vi "CSGaussmeterGUI.panel.vi"() -> ()   [LabVIEW 2014, in "CSGaussmeterGUI.lvlib"]
doc: "This is the VI template for the Gaussmeter class."
uses:
  CSGaussmeterGUI.lvlib
  instr.lib/FH_55/TypeDef/Display.ctl
  instr.lib/FH_55/TypeDef/Unit.ctl
  instr.lib/FH_55/TypeDef/Temp_Unit.ctl
  instr.lib/FH_55/TypeDef/Max.ctl
  instr.lib/FH_55/TypeDef/Range.ctl
  instr.lib/FH_55/TypeDef/Unit2.ctl
  CS_Core/CSSystem/CoreDefs/CoreDefs.rawDataType.ctl
  CS_Core/CSSystem/CoreLib/CoreLib.short 2 byte array.vi
  CS_Core/CSSystem/CoreLib/CoreLib.double 2 byte array.vi
  CS_Core/CSSystem/CoreLib/CoreLib.string 2 byte array.vi
  CSGaussmeter/CSGaussmeter.lvlib
  CS_Core/CSSystem/CoreLib/CoreLib.lvlib
  CS_Core/BaseProcess/BaseProcess.lvlib
  CS_Core/CSSystem/CSSystemLib/CSSystemLib.lvlib
  CSlibraries/UtilityLib/UtilityLib.lvlib
  CS_Core/CSObj/CSObj.lvlib
  CS_Core/GUIs/GOGUserGUIs/DeviceBaseGUI/DeviceBaseGUI.lvlib
  instr.lib/FH_55/FH 55.lvlib
panel:
  in  "object ref":refnum<vi>
  out "Messwerte 2":string
  out "status abc":string
  out "status TF":bool
  in  "Stop":bool
  in  "Lesen":bool
  in  "Cluster":cluster{"String":string, "byteArray":T1}
  in  "error out 2":errorcluster
  in  "Control":T7 {"Lower"."Numeric" format="%#_4f"; "Set_Rel"."Numeric" format="%#_4f"; "UPPER"."Numeric" format="%#_4f"}
  in  "Messwerte":cluster{"Numeric":i32, "OK Button":bool}={"Numeric"=1, "OK Button"=FALSE} {"Numeric" min=1}
  out "FH 55 Gauss-/Teslameter":T8
  out "error out":errorcluster
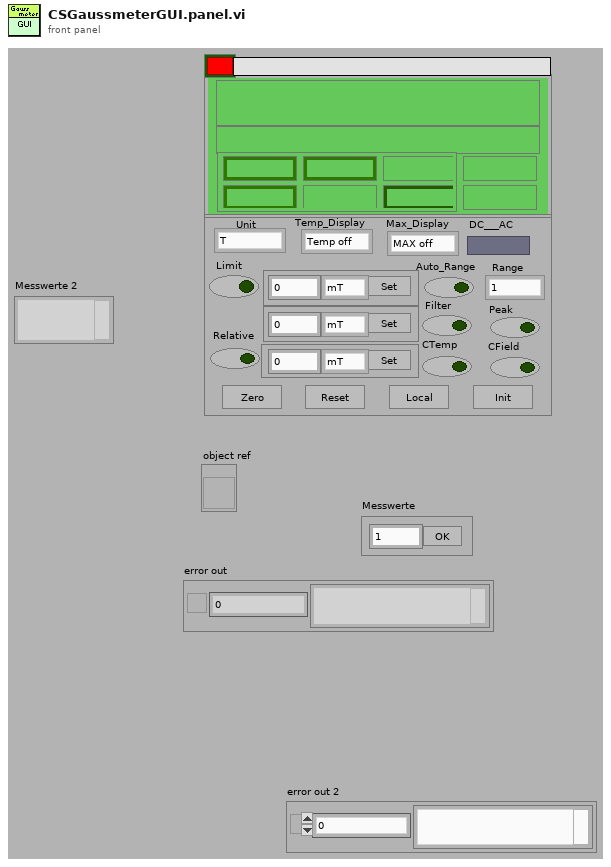
[diagram p1: front panel]
types:
  T1 = typedef "CoreDefs.rawDataType.ctl" = i8[]
  T2 = typedef "FH 55.lvlib/Unit.ctl" = enum16{"T", "G", "A/m"}
  T3 = typedef "FH 55.lvlib/Temp_Unit.ctl" = enum16{"Temp off", "Celsius", "Fahrenheit"}
  T4 = typedef "FH 55.lvlib/Max.ctl" = enum16{"MAX off", "Show MAX", "MAX/MIN"}
  T5 = typedef "FH 55.lvlib/Range.ctl" = enum16{"1", "2", "3", "4", "5", "6", "7"}
  T6 = typedef "FH 55.lvlib/Unit2.ctl" = enum16{"mT", "G", "kA/m"}
  T7 = cluster{" Limit":bool, "Unit":T2, "Temp_Display":T3, "Max_Display":T4, " Filter":bool, " Peak":bool, " Auto_Range":bool, "Range":T5, " Relative":bool, " CTemp":bool, " CField":bool, "DC___AC ":bool, "Lower":cluster{"Numeric":dbl, "Cancel Button":bool, "Unit":T6}, "UPPER":cluster{"Numeric":dbl, "Cancel Button":bool, "Unit":T6}, "Set_Rel":cluster{"Numeric":dbl, "Cancel Button":bool, "Unit":T6}, "Zero":bool, "Reset":bool, " Local":bool, "Init ":bool}
  T8 = typedef "FH 55.lvlib/Display.ctl" = cluster{"current value":string, "Limit":string, "Remote":string, "function ":string, "Cluster":cluster{"AC/DC":string, "Auto":string, "Filter":string, "Range":string, "Rel":string, "Peak":string}}
  T9 = typedef "DeviceBaseGUI.lvlib/DeviceBaseGUI.i attribute.ctl" = cluster{"GOGFrontPanel.i attribute":T10}
  T10 = typedef "GOGFrontPanel.lvlib/GOGFrontPanel.i attribute.ctl" = cluster{"GOGObject":string, "Object":string, "Method":string, "Descriptor":T11, "Input Descriptor":string, "Output Descriptor":string, "inputNames":string[], "outputNames":string[], "Values":cluster{"descriptor":string, "value":string}[]}
  T11 = typedef "BaseProcess.lvlib/BaseProcess.descriptor string definition.ctl" = string
  T12 = typedef "CSGaussmeter.lvlib/CSGaussmeter.i attribute.ctl" = cluster{"Name":string, "VISA Resource Name":refnum<visa-resource-name>, "actValues":cluster{" Limit":bool, "Unit ":T2, "Temp_Unit":T3, "Max":T4, " Filter":bool, " Peak":bool, " Auto_Range":bool, "Range":T5, " Rel":bool, " CTemp":bool, " CField":bool, "AC_DC ":bool, "Set_lower":cluster{"Numeric":dbl, "Cancel Button":bool, "Unit":T6}, "Set_upper":cluster{"Numeric":dbl, "Cancel Button":bool, "Unit":T6}, "Set_Rel":cluster{"Numeric":dbl, "Cancel Button":bool, "Unit":T6}, "Zero":bool, " Local":bool, "Reset":bool, " Init":bool}, "FH 55 Gauss-/Teslameter":T8, "MAX_Value":T13, "MIN_Value":T13, "Rel_Value":T13, "Array ":string[], "LIMU":dbl, " LIML":dbl, "Messwerte 2":string, "Messwerte ":cluster{"Numeric":i32, "OK Button":bool}, "serviceID":cluster{"Current ID":i32, "Unit ID":i32, "Temp ID":i32, "Name ID \n":i32, "Visa ID ":i32}, "setValues ":cluster{" Limit":bool, "Unit ":T2, "Temp_Unit":T3, "Max":T4, " Filter":bool, " Peak":bool, " Auto_Range":bool, "Range":T5, " Rel":bool, " CTemp":bool, " CField":bool, "AC_DC ":bool, "Set_lower":cluster{"Numeric":dbl, "Cancel Button":bool, "Unit":T6}, "Set_upper":cluster{"Numeric":dbl, "Cancel Button":bool, "Unit":T6}, "Set_Rel":cluster{"Numeric":dbl, "Cancel Button":bool, "Unit":T6}, "Zero":bool, " Local":bool, "Reset":bool, " Init":bool}}
  T13 = typedef "FH 55.lvlib/Value_String.ctl" = cluster{"Numeric":dbl, "String":string}
  T14 = cluster{" Limit":bool, "Unit ":T2, "Temp_Unit":T3, "Max":T4, " Filter":bool, " Peak":bool, " Auto_Range":bool, "Range":T5, " Rel":bool, " CTemp":bool, " CField":bool, "AC_DC ":bool, "Set_lower":cluster{"Numeric":dbl, "Cancel Button":bool, "Unit":T6}, "Set_upper":cluster{"Numeric":dbl, "Cancel Button":bool, "Unit":T6}, "Set_Rel":cluster{"Numeric":dbl, "Cancel Button":bool, "Unit":T6}, "Zero":bool, " Local":bool, "Reset":bool, " Init":bool}
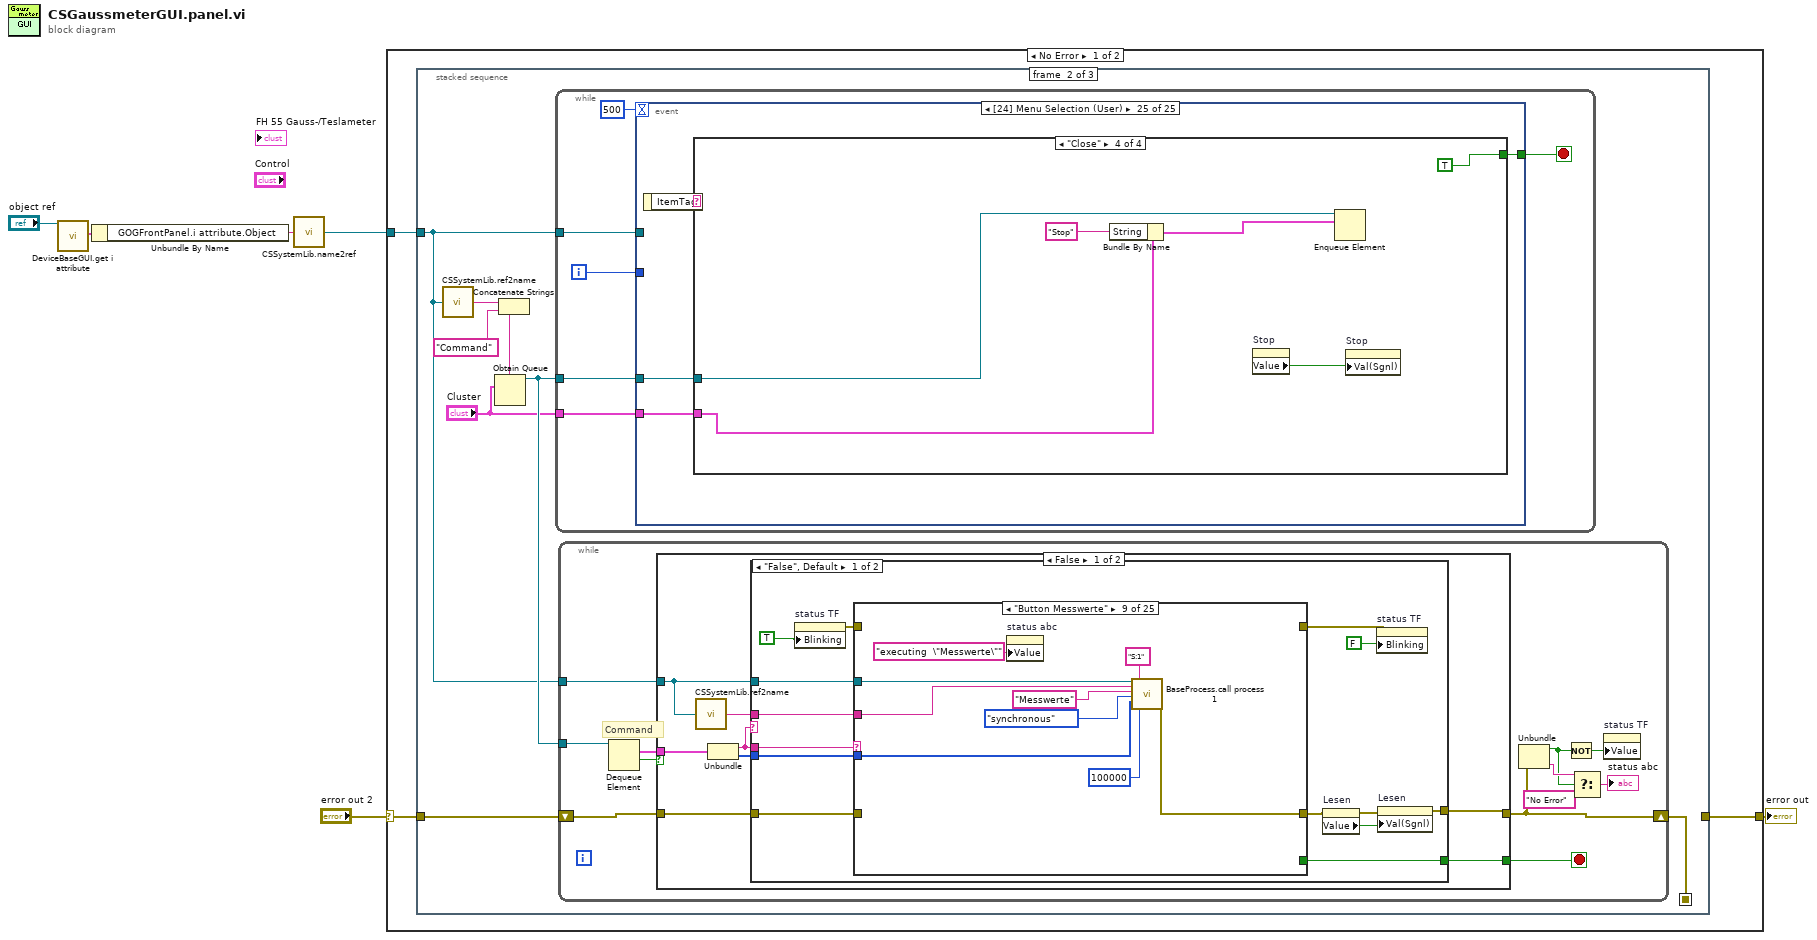
[diagram p0: block diagram]
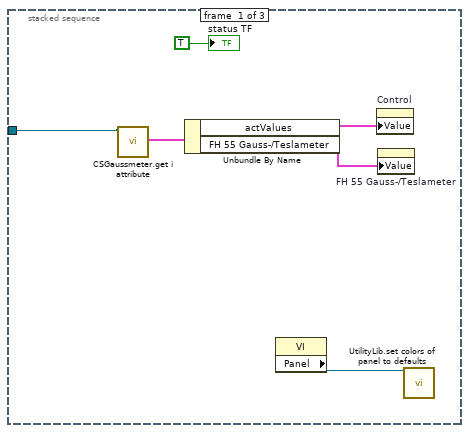
[diagram p2: hidden frame]
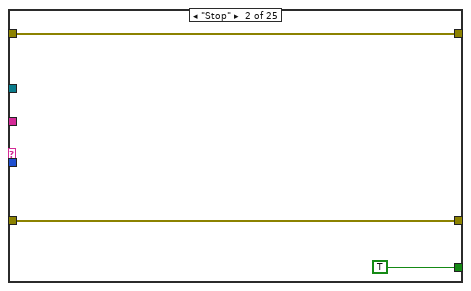
[diagram p4: hidden frame]
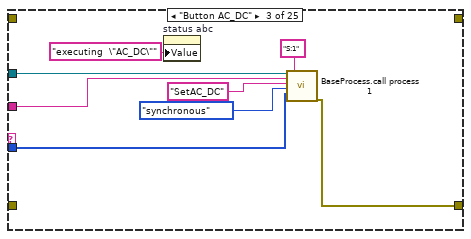
[diagram p5: hidden frame]
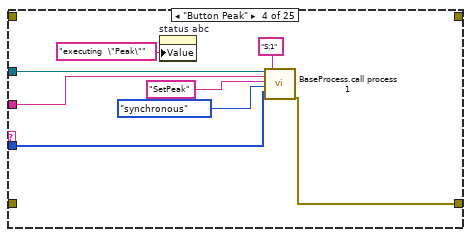
[diagram p6: hidden frame]
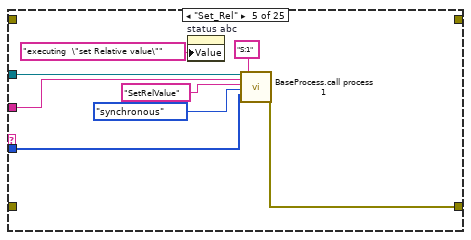
[diagram p7: hidden frame]
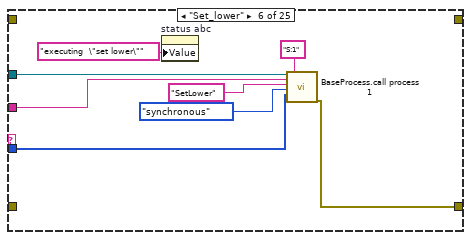
[diagram p8: hidden frame]
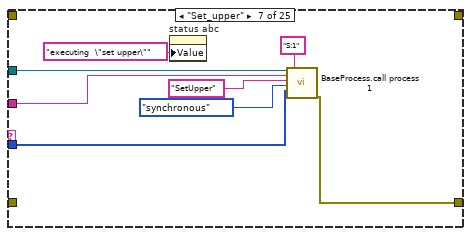
[diagram p9: hidden frame]
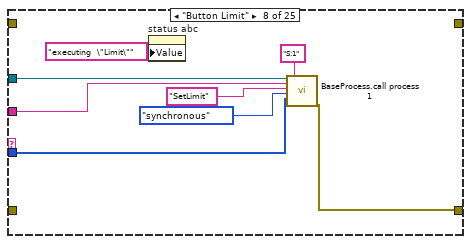
[diagram p10: hidden frame]
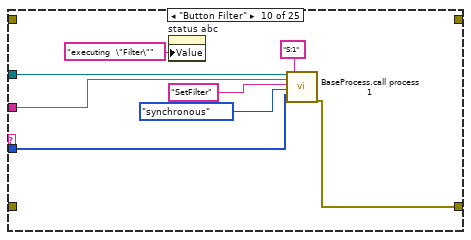
[diagram p11: hidden frame]
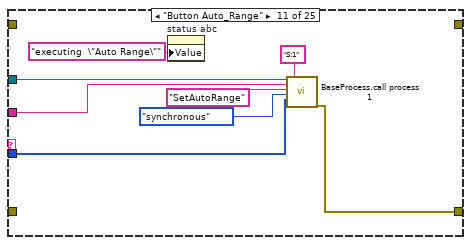
[diagram p12: hidden frame]
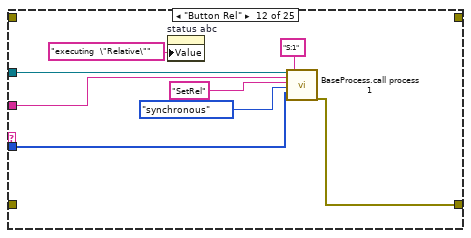
[diagram p13: hidden frame]
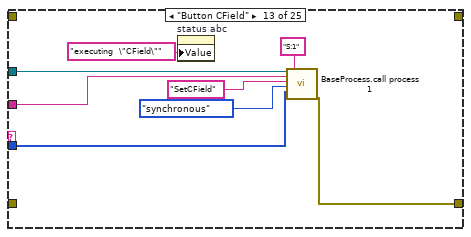
[diagram p14: hidden frame]
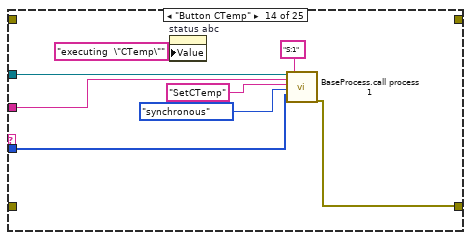
[diagram p15: hidden frame]
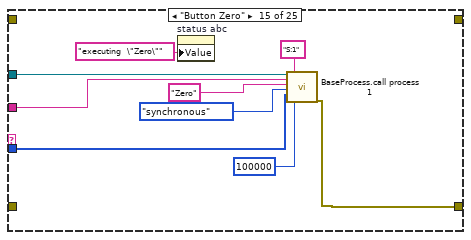
[diagram p16: hidden frame]
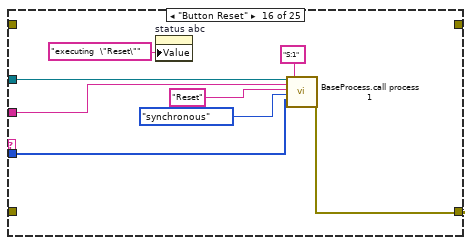
[diagram p17: hidden frame]
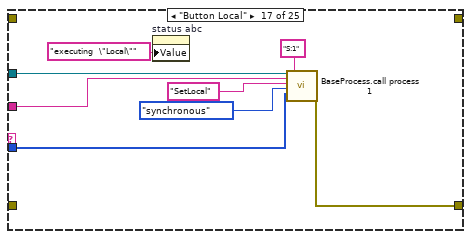
[diagram p18: hidden frame]
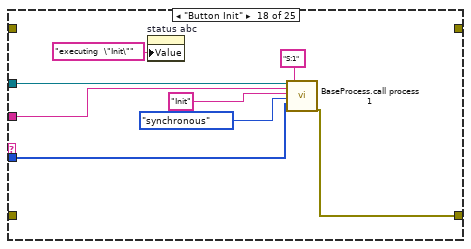
[diagram p19: hidden frame]
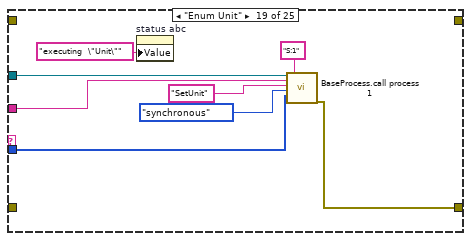
[diagram p20: hidden frame]
diagram:
  n1 = call "DeviceBaseGUI.get i attribute.vi"("i ref in"="object ref") -> ("i attribute"=w3:T9)  [unwired: 16 in, 2 out]
  n2 = Unbundle By Name(w3) -> ("GOGFrontPanel.i attribute.Object"=w2:string)
  n3 = call "CSSystemLib.name2ref.vi"("name"=w2) -> ("obj refnum"=w1:refnum<vi>)
  n4 = case shown="No Error" "error out 2" {
    selector: "error out 2" -> [w9 w521]
    tunnel: [w7 w521] -> w6
    tunnel: w1 -> [w8 _]
    frame No Error {
      n5 = stacked-sequence {
        seq-local: [_ w20 _] -> [_ _ w502]
        tunnel: w9 -> [_ w22 _]
        tunnel: w8 -> [w14 w19 w503]
        tunnel: [_ _ w501] -> w7
        frame #0 {
          n6 = call "CSGaussmeter.get i attribute.vi"("i ref in"=w14) -> ("i attribute"=w13:T12)  [unwired: 16 in, 2 out]
          n7 = Unbundle By Name(w13) -> ("actValues"=w10:T14, "FH 55 Gauss-/Teslameter"=w15:T8)
          n8 = property on="Property Node" class="VI"() -> ("Panel"=w12:refnum<vi>)  [unwired: 2 in, 2 out]
          n9 = property on="Control" class="Clust (strict)"("Value"=w10) -> ()  [unwired: 2 in, 2 out]
          n10 = property on="FH 55 Gauss-/Teslameter" class="Clust (strict)"("Value"=w15) -> ()  [unwired: 2 in, 2 out]
          n11 = call "UtilityLib.set colors of panel to defaults.vi"("Front Panel"=w12) -> ()  [unwired: 18 in, 1 out]
          "status TF" <- TRUE ("status TF")
        }
        frame #1 {
          n12 = call "CSSystemLib.ref2name.vi"("obj refnum"=w19) -> ("name"=w18:string)
          n13 = Concatenate Strings(w18, "Command" ("name (unnamed)")) -> (w16:string)
          n14 = Obtain Queue(name (unnamed)=w16, element data type="Cluster") -> (queue out=w23:refnum<queue>)  [unwired: 3 in, 2 out]
          n15 = while {
            tunnel: w23 -> [w271]
            tunnel: "Cluster" -> [w270]
            tunnel: w19 -> [w269]
            i -> [w267]
            stop <- w268 stop-if-true
            n16 = event shown="[24] Menu Selection (User)" {
              selector: _ -> [_ _ _ _ _ _ _ _ _ _ _ _ _ _ _ _ _ _ _ _ _ _ _ _ _]
              dyn-events: _ -> [_ _ _ _ _ _ _ _ _ _ _ _ _ _ _ _ _ _ _ _ _ _ _ _ _]
              timeout: 500 -> [_ _ _ _ _ _ _ _ _ _ _ _ _ _ _ _ _ _ _ _ _ _ _ _ _]
              tunnel: w271 -> [_ w298 w304 w309 w319 w327 w336 w345 w355 w362 w371 w380 w389 w398 w407 w416 w423 w430 w437 w444 w450 w456 w462 w468 w474]
              tunnel: w270 -> [_ w299 w305 w310 w318 w328 w337 w346 w354 w361 w370 w379 w388 w397 w406 w415 w422 w429 w436 w443 w449 w455 w461 w467 w473]
              tunnel: w269 -> [w276 _ _ _ _ _ _ _ _ _ _ _ _ _ _ _ _ _ _ _ _ _ _ _ _]
              tunnel: [_ _ _ TRUE _ _ _ _ _ _ _ _ _ _ _ _ _ _ _ _ _ _ _ _ w471] -> w268
              tunnel: w267 -> [w275 _ _ _ _ _ _ _ _ _ _ _ _ _ _ _ _ _ _ _ _ _ _ _ _]
              event Timeout {
                n17 = event-data() -> ()  [unwired: 1 in, 1 out]
                n18 = Quotient & Remainder(x=w275, y=100000000) -> (x-y*floor(x/y)=w273:i32)  [unwired: 1 out]
                n19 = case shown="Default" w273 {
                  tunnel: w276 -> [w281 w291]
                  frame Default {
                    n20 = call "CSGaussmeter.get i attribute.vi"("i ref in"=w281) -> ("i attribute"=w280:T12)  [unwired: 16 in, 2 out]
                    n21 = Unbundle By Name(w280) -> ("FH 55 Gauss-/Teslameter"=w277:T8, "FH 55 Gauss-/Teslameter.Limit"=w279:string, "actValues.Limit"=w278:bool)
                    n22 = case shown="True" w278 {
                      tunnel: w279 -> [_ w283]
                      frame False {
                        n23 = property on="Limit" class="Str"("Blinking"=FALSE) -> ()  [unwired: 2 in, 2 out]
                      }
                      frame True {
                        n24 = case shown="\"OK\"" w283 {
                          frame "OK" {
                            n25 = property on="Limit" class="Str"("Blinking"=FALSE) -> ()  [unwired: 2 in, 2 out]
                          }
                          frame Default {
                            n26 = property on="Limit" class="Str"("Blinking"=TRUE) -> ()  [unwired: 2 in, 2 out]
                          }
                        }
                      }
                    }
                    n27 = property on="FH 55 Gauss-/Teslameter" class="Clust (strict)"("Value"=w277) -> ()  [unwired: 2 in, 2 out]
                  }
                  frame 0 {
                    n28 = call "CSGaussmeter.get i attribute.vi"("i ref in"=w291) -> ("i attribute"=w290:T12)  [unwired: 16 in, 2 out]
                    n29 = Unbundle By Name(w290) -> ("actValues"=w286:T14, "FH 55 Gauss-/Teslameter"=w287:T8, "FH 55 Gauss-/Teslameter.Limit"=w289:string, "actValues.Limit"=w288:bool)
                    n30 = case shown="True" w288 {
                      tunnel: w289 -> [_ w293]
                      frame False {
                        n31 = property on="Limit" class="Str"("Blinking"=FALSE) -> ()  [unwired: 2 in, 2 out]
                      }
                      frame True {
                        n32 = case shown="Default" w293 {
                          frame "OK" {
                            n33 = property on="Limit" class="Str"("Blinking"=FALSE) -> ()  [unwired: 2 in, 2 out]
                          }
                          frame Default {
                            n34 = property on="Limit" class="Str"("Blinking"=TRUE) -> ()  [unwired: 2 in, 2 out]
                          }
                        }
                      }
                    }
                    n35 = property on="Control" class="Clust (strict)"("Value"=w286) -> ()  [unwired: 2 in, 2 out]
                    n36 = property on="FH 55 Gauss-/Teslameter" class="Clust (strict)"("Value"=w287) -> ()  [unwired: 2 in, 2 out]
                  }
                }
              }
              event "status TF": Key Down {
                n37 = event-data() -> ()  [unwired: 1 in, 10 out]
                n38 = call-poly "CoreLib.data 2 byte array.vi"("i16"=i16 0) -> ("byteArray out"=w297:T1)  [unwired: 18 in]
                n39 = Bundle By Name(cluster=w299, "String"="Button OK" ("command"), "byteArray"=w297) -> (w300:cluster{"String":string, "byteArray":T1})
                n40 = Enqueue Element(queue=w298, element=w300) -> ()  [unwired: 2 in, 3 out]
              }
              event "Lesen": Value Change {
                n41 = event-data() -> ()  [unwired: 1 in, 6 out]
                n42 = call-poly "CoreLib.data 2 byte array.vi"("i16"=i16 0) -> ("byteArray out"=w303:T1)  [unwired: 18 in]
                n43 = Bundle By Name(cluster=w305, "String"="Lesen" ("command"), "byteArray"=w303) -> (w306:cluster{"String":string, "byteArray":T1})
                n44 = Enqueue Element(queue=w304, element=w306) -> ()  [unwired: 2 in, 3 out]
              }
              event "Stop": Value Change; Panel Close; Application Instance Close {
                n45 = event-data() -> ()  [unwired: 1 in, 1 out]
                n46 = Bundle By Name(cluster=w310, "String"="Stop" ("command")) -> (w311:cluster{"String":string, "byteArray":T1})
                n47 = Enqueue Element(queue=w309, element=w311) -> ()  [unwired: 2 in, 3 out]
              }
              event "Control.Peak": Value Change {
                n48 = event-data() -> ("NewVal"=w314:bool)  [unwired: 1 in]
                n49 = Select(t=i16 1, s=w314, f=i16 0) -> (s? t:f=w313:i16)
                n50 = call-poly "CoreLib.data 2 byte array.vi"("i16"=w313) -> ("byteArray out"=w317:T1)  [unwired: 18 in]
                n51 = Bundle By Name(cluster=w318, "String"="Button Peak" ("command"), "byteArray"=w317) -> (w320:cluster{"String":string, "byteArray":T1})
                n52 = Enqueue Element(queue=w319, element=w320) -> ()  [unwired: 2 in, 3 out]
              }
              event "Control.Set_Rel.Cancel Button": Value Change {
                n53 = event-data() -> ("OldVal"=w326:bool)  [unwired: 1 in]
                n54 = property on="Cancel Button" class="Bool (strict)"("Value"=w326) -> ()  [unwired: 2 in, 2 out]
                n55 = property on="Unit" class="Enum (strict)"() -> ("Value"=w322:T6)  [unwired: 2 in, 2 out]
                n56 = property on="Numeric" class="DigNum (strict)"() -> ("Value"=w323:dbl)  [unwired: 2 in, 2 out]
                n57 = call-poly "CoreLib.data 2 byte array.vi"("f64"=w323) -> ("byteArray out"=w324:T1)  [unwired: 18 in]
                n58 = call-poly "CoreLib.data 2 byte array.vi"("byteArray"=w324, "i16"=w322) -> ("byteArray out"=w325:T1)  [unwired: 17 in]
                n59 = Bundle By Name(cluster=w328, "String"="Set_Rel" ("command"), "byteArray"=w325) -> (w329:cluster{"String":string, "byteArray":T1})
                n60 = Enqueue Element(queue=w327, element=w329) -> ()  [unwired: 2 in, 3 out]
              }
              event "Control.Lower.Cancel Button": Value Change {
                n61 = event-data() -> ("OldVal"=w335:bool)  [unwired: 1 in]
                n62 = property on="Numeric" class="DigNum (strict)"() -> ("Value"=w332:dbl)  [unwired: 2 in, 2 out]
                n63 = property on="Unit" class="Enum (strict)"() -> ("Value"=w331:T6)  [unwired: 2 in, 2 out]
                n64 = property on="Cancel Button" class="Bool (strict)"("Value"=w335) -> ()  [unwired: 2 in, 2 out]
                n65 = call-poly "CoreLib.data 2 byte array.vi"("f64"=w332) -> ("byteArray out"=w334:T1)  [unwired: 18 in]
                n66 = call-poly "CoreLib.data 2 byte array.vi"("byteArray"=w334, "i16"=w331) -> ("byteArray out"=w333:T1)  [unwired: 17 in]
                n67 = Bundle By Name(cluster=w337, "String"="Set_lower" ("command"), "byteArray"=w333) -> (w338:cluster{"String":string, "byteArray":T1})
                n68 = Enqueue Element(queue=w336, element=w338) -> ()  [unwired: 2 in, 3 out]
              }
              event "Control.UPPER.Cancel Button": Value Change {
                n69 = event-data() -> ("OldVal"=w344:bool)  [unwired: 1 in]
                n70 = property on="Numeric" class="DigNum (strict)"() -> ("Value"=w341:dbl)  [unwired: 2 in, 2 out]
                n71 = property on="Unit" class="Enum (strict)"() -> ("Value"=w340:T6)  [unwired: 2 in, 2 out]
                n72 = property on="Cancel Button" class="Bool (strict)"("Value"=w344) -> ()  [unwired: 2 in, 2 out]
                n73 = call-poly "CoreLib.data 2 byte array.vi"("f64"=w341) -> ("byteArray out"=w343:T1)  [unwired: 18 in]
                n74 = call-poly "CoreLib.data 2 byte array.vi"("byteArray"=w343, "i16"=w340) -> ("byteArray out"=w342:T1)  [unwired: 17 in]
                n75 = Bundle By Name(cluster=w346, "String"="Set_upper" ("command"), "byteArray"=w342) -> (w347:cluster{"String":string, "byteArray":T1})
                n76 = Enqueue Element(queue=w345, element=w347) -> ()  [unwired: 2 in, 3 out]
              }
              event "Control.Limit": Value Change {
                n77 = event-data() -> ("NewVal"=w350:bool)  [unwired: 1 in]
                n78 = Select(t=i16 1, s=w350, f=i16 0) -> (s? t:f=w349:i16)
                n79 = call-poly "CoreLib.data 2 byte array.vi"("i16"=w349) -> ("byteArray out"=w353:T1)  [unwired: 18 in]
                n80 = Bundle By Name(cluster=w354, "String"="Button Limit" ("command"), "byteArray"=w353) -> (w356:cluster{"String":string, "byteArray":T1})
                n81 = Enqueue Element(queue=w355, element=w356) -> ()  [unwired: 2 in, 3 out]
              }
              event "Messwerte.OK Button": Value Change {
                n82 = event-data() -> ("OldVal"=w360:bool)  [unwired: 1 in]
                n83 = property on="Numeric" class="DigNum (strict)"() -> ("Value"=w358:i32)  [unwired: 2 in, 2 out]
                n84 = property on="OK Button" class="Bool (strict)"("Value"=w360) -> ()  [unwired: 2 in, 2 out]
                n85 = call-poly "CoreLib.data 2 byte array.vi"("i16"=w358) -> ("byteArray out"=w359:T1)  [unwired: 18 in]
                n86 = Bundle By Name(cluster=w361, "String"="Button Messwerte" ("command"), "byteArray"=w359) -> (w363:cluster{"String":string, "byteArray":T1})
                n87 = Enqueue Element(queue=w362, element=w363) -> ()  [unwired: 2 in, 3 out]
              }
              event "Control.Filter": Value Change {
                n88 = event-data() -> ("NewVal"=w367:bool)  [unwired: 1 in]
                n89 = Select(t=i16 1, s=w367, f=i16 0) -> (s? t:f=w365:i16)
                n90 = call-poly "CoreLib.data 2 byte array.vi"("i16"=w365) -> ("byteArray out"=w366:T1)  [unwired: 18 in]
                n91 = Bundle By Name(cluster=w370, "String"="Button Filter" ("command"), "byteArray"=w366) -> (w372:cluster{"String":string, "byteArray":T1})
                n92 = Enqueue Element(queue=w371, element=w372) -> ()  [unwired: 2 in, 3 out]
              }
              event "Control.Auto_Range": Value Change {
                n93 = event-data() -> ("NewVal"=w377:bool)  [unwired: 1 in]
                n94 = Select(t=i16 1, s=w377, f=i16 0) -> (s? t:f=w374:i16)
                n95 = call-poly "CoreLib.data 2 byte array.vi"("i16"=w374) -> ("byteArray out"=w375:T1)  [unwired: 18 in]
                n96 = Bundle By Name(cluster=w379, "String"="Button Auto_Range" ("command"), "byteArray"=w375) -> (w381:cluster{"String":string, "byteArray":T1})
                n97 = Enqueue Element(queue=w380, element=w381) -> ()  [unwired: 2 in, 3 out]
              }
              event "Control.Relative": Value Change {
                n98 = event-data() -> ("NewVal"=w385:bool)  [unwired: 1 in]
                n99 = Select(t=i16 1, s=w385, f=i16 0) -> (s? t:f=w383:i16)
                n100 = call-poly "CoreLib.data 2 byte array.vi"("i16"=w383) -> ("byteArray out"=w384:T1)  [unwired: 18 in]
                n101 = Bundle By Name(cluster=w388, "String"="Button Rel" ("command"), "byteArray"=w384) -> (w390:cluster{"String":string, "byteArray":T1})
                n102 = Enqueue Element(queue=w389, element=w390) -> ()  [unwired: 2 in, 3 out]
              }
              event "Control.CField": Value Change {
                n103 = event-data() -> ("NewVal"=w395:bool)  [unwired: 1 in]
                n104 = Select(t=i16 1, s=w395, f=i16 0) -> (s? t:f=w392:i16)
                n105 = call-poly "CoreLib.data 2 byte array.vi"("i16"=w392) -> ("byteArray out"=w393:T1)  [unwired: 18 in]
                n106 = Bundle By Name(cluster=w397, "String"="Button CField" ("command"), "byteArray"=w393) -> (w399:cluster{"String":string, "byteArray":T1})
                n107 = Enqueue Element(queue=w398, element=w399) -> ()  [unwired: 2 in, 3 out]
              }
              event "Control.CTemp": Value Change {
                n108 = event-data() -> ("NewVal"=w403:bool)  [unwired: 1 in]
                n109 = Select(t=i16 1, s=w403, f=i16 0) -> (s? t:f=w401:i16)
                n110 = call-poly "CoreLib.data 2 byte array.vi"("i16"=w401) -> ("byteArray out"=w402:T1)  [unwired: 18 in]
                n111 = Bundle By Name(cluster=w406, "String"="Button CTemp" ("command"), "byteArray"=w402) -> (w408:cluster{"String":string, "byteArray":T1})
                n112 = Enqueue Element(queue=w407, element=w408) -> ()  [unwired: 2 in, 3 out]
              }
              event "Control.DC___AC": Value Change {
                n113 = event-data() -> ("NewVal"=w411:bool)  [unwired: 1 in]
                n114 = Select(t=i16 1, s=w411, f=i16 0) -> (s? t:f=w410:i16)
                n115 = call-poly "CoreLib.data 2 byte array.vi"("i16"=w410) -> ("byteArray out"=w412:T1)  [unwired: 18 in]
                n116 = Bundle By Name(cluster=w415, "String"="Button AC_DC" ("command"), "byteArray"=w412) -> (w417:cluster{"String":string, "byteArray":T1})
                n117 = Enqueue Element(queue=w416, element=w417) -> ()  [unwired: 2 in, 3 out]
              }
              event "Control.Zero": Value Change {
                n118 = event-data() -> ("OldVal"=w420:bool)  [unwired: 1 in]
                n119 = property on="Zero" class="Bool (strict)"("Value"=w420) -> ()  [unwired: 2 in, 2 out]
                n120 = call-poly "CoreLib.data 2 byte array.vi"("i16"=i16 0) -> ("byteArray out"=w421:T1)  [unwired: 18 in]
                n121 = Bundle By Name(cluster=w422, "String"="Button Zero" ("command"), "byteArray"=w421) -> (w424:cluster{"String":string, "byteArray":T1})
                n122 = Enqueue Element(queue=w423, element=w424) -> ()  [unwired: 2 in, 3 out]
              }
              event "Control.Reset": Value Change {
                n123 = event-data() -> ("OldVal"=w427:bool)  [unwired: 1 in]
                n124 = property on="Reset" class="Bool (strict)"("Value"=w427) -> ()  [unwired: 2 in, 2 out]
                n125 = call-poly "CoreLib.data 2 byte array.vi"("i16"=i16 0) -> ("byteArray out"=w428:T1)  [unwired: 18 in]
                n126 = Bundle By Name(cluster=w429, "String"="Button Reset" ("command"), "byteArray"=w428) -> (w431:cluster{"String":string, "byteArray":T1})
                n127 = Enqueue Element(queue=w430, element=w431) -> ()  [unwired: 2 in, 3 out]
              }
              event "Control.Local": Value Change {
                n128 = event-data() -> ("OldVal"=w434:bool)  [unwired: 1 in]
                n129 = property on="Local" class="Bool (strict)"("Value"=w434) -> ()  [unwired: 2 in, 2 out]
                n130 = call-poly "CoreLib.data 2 byte array.vi"("i16"=i16 0) -> ("byteArray out"=w435:T1)  [unwired: 18 in]
                n131 = Bundle By Name(cluster=w436, "String"="Button Local" ("command"), "byteArray"=w435) -> (w438:cluster{"String":string, "byteArray":T1})
                n132 = Enqueue Element(queue=w437, element=w438) -> ()  [unwired: 2 in, 3 out]
              }
              event "Control.Init": Value Change {
                n133 = event-data() -> ("OldVal"=w441:bool)  [unwired: 1 in]
                n134 = property on="Init" class="Bool (strict)"("Value"=w441) -> ()  [unwired: 2 in, 2 out]
                n135 = call-poly "CoreLib.data 2 byte array.vi"("i16"=i16 0) -> ("byteArray out"=w442:T1)  [unwired: 18 in]
                n136 = Bundle By Name(cluster=w443, "String"="Button Init" ("command"), "byteArray"=w442) -> (w445:cluster{"String":string, "byteArray":T1})
                n137 = Enqueue Element(queue=w444, element=w445) -> ()  [unwired: 2 in, 3 out]
              }
              event Value Change {
                n138 = event-data() -> ("NewVal"=w447:T2)  [unwired: 1 in]
                n139 = call-poly "CoreLib.data 2 byte array.vi"("i16"=w447) -> ("byteArray out"=w448:T1)  [unwired: 18 in]
                n140 = Bundle By Name(cluster=w449, "String"="Enum Unit" ("command"), "byteArray"=w448) -> (w451:cluster{"String":string, "byteArray":T1})
                n141 = Enqueue Element(queue=w450, element=w451) -> ()  [unwired: 2 in, 3 out]
              }
              event Value Change {
                n142 = event-data() -> ("NewVal"=w453:T5)  [unwired: 1 in]
                n143 = call-poly "CoreLib.data 2 byte array.vi"("i16"=w453) -> ("byteArray out"=w454:T1)  [unwired: 18 in]
                n144 = Bundle By Name(cluster=w455, "String"="Enum Range" ("command"), "byteArray"=w454) -> (w457:cluster{"String":string, "byteArray":T1})
                n145 = Enqueue Element(queue=w456, element=w457) -> ()  [unwired: 2 in, 3 out]
              }
              event Value Change {
                n146 = event-data() -> ("NewVal"=w459:T4)  [unwired: 1 in]
                n147 = call-poly "CoreLib.data 2 byte array.vi"("i16"=w459) -> ("byteArray out"=w460:T1)  [unwired: 18 in]
                n148 = Bundle By Name(cluster=w461, "String"="Enum Max" ("command"), "byteArray"=w460) -> (w463:cluster{"String":string, "byteArray":T1})
                n149 = Enqueue Element(queue=w462, element=w463) -> ()  [unwired: 2 in, 3 out]
              }
              event Value Change {
                n150 = event-data() -> ("NewVal"=w465:T3)  [unwired: 1 in]
                n151 = call-poly "CoreLib.data 2 byte array.vi"("i16"=w465) -> ("byteArray out"=w466:T1)  [unwired: 18 in]
                n152 = Bundle By Name(cluster=w467, "String"="Enum Temp" ("command"), "byteArray"=w466) -> (w469:cluster{"String":string, "byteArray":T1})
                n153 = Enqueue Element(queue=w468, element=w469) -> ()  [unwired: 2 in, 3 out]
              }
              event Menu Selection (User) {
                n154 = event-data() -> ("ItemTag"=w472:string)  [unwired: 1 in]
                n155 = case shown="\"Close\"" w472 {
                  selector: w472 -> [_ w477 w487 _]
                  tunnel: w474 -> [_ w483 w493 w497]
                  tunnel: w473 -> [_ w482 w492 w496]
                  tunnel: [_ _ _ TRUE] -> w471
                  frame "False", Default {
                  }
                  frame "SaveSettings" {
                    n156 = String To Path(string="F:\\LVSCC\\LV820\\GPL\\Projects\\cs-framework\\CSClass\\CSHitrap\\CSGaussmeter\\settings\\") -> (path=w475:path)
                    n157 = File Dialog(7:"setting file" ("prompt"), 11:w475) -> (3:w479:path)  [unwired: 5 in, 3 out]
                    n158 = Path To String(path=w479) -> (string=w478:string)
                    n159 = call-poly "CoreLib.data 2 byte array.vi"("string"=w478) -> ("byteArray out"=w481:T1)  [unwired: 18 in]
                    n160 = Bundle By Name(cluster=w482, "String"=w477, "byteArray"=w481) -> (w484:cluster{"String":string, "byteArray":T1})
                    n161 = Enqueue Element(queue=w483, element=w484) -> ()  [unwired: 2 in, 3 out]
                  }
                  frame "LoadSettings" {
                    n162 = String To Path(string="F:\\LVSCC\\LV820\\GPL\\Projects\\cs-framework\\CSClass\\CSHitrap\\CSGaussmeter\\settings\\") -> (path=w486:path)
                    n163 = File Dialog(7:"load file" ("prompt"), 11:w486) -> (3:w489:path)  [unwired: 5 in, 3 out]
                    n164 = Path To String(path=w489) -> (string=w488:string)
                    n165 = call-poly "CoreLib.data 2 byte array.vi"("string"=w488) -> ("byteArray out"=w491:T1)  [unwired: 18 in]
                    n166 = Bundle By Name(cluster=w492, "String"=w487, "byteArray"=w491) -> (w494:cluster{"String":string, "byteArray":T1})
                    n167 = Enqueue Element(queue=w493, element=w494) -> ()  [unwired: 2 in, 3 out]
                  }
                  frame "Close" {
                    n168 = Bundle By Name(cluster=w496, "String"="Stop" ("command")) -> (w498:cluster{"String":string, "byteArray":T1})
                    n169 = property on="Stop" class="Bool (strict)"() -> ("Value"=w500:bool)  [unwired: 2 in, 2 out]
                    n170 = Enqueue Element(queue=w497, element=w498) -> ()  [unwired: 2 in, 3 out]
                    n171 = property on="Stop" class="Bool (strict)"("Val(Sgnl)"=w500) -> ()  [unwired: 2 in, 2 out]
                  }
                }
              }
            }
          }
          n172 = while {
            tunnel: w23 -> [w35]
            shift-right: [w31] -> w20
            shift-left: w22 -> [w32]
            tunnel: w19 -> [w30]
            stop <- w29 stop-if-true
            # "Command"
            n173 = Dequeue Element(queue=w35) -> (element=w33:cluster{"String":string, "byteArray":T1}, timed out?=w34:bool)  [unwired: 2 in, 2 out]
            n174 = case shown="False" w34 {
              tunnel: w33 -> [w43 _]
              tunnel: w32 -> [w41 w266]
              tunnel: [w37 w266] -> w31
              tunnel: w30 -> [w40 _]
              tunnel: [w38 FALSE ("Boolean")] -> w29
              frame False {
                n175 = call "CSSystemLib.ref2name.vi"("obj refnum"=w40) -> ("name"=w39:string)
                n176 = Unbundle(w43) -> ("String"=w36:string, "byteArray"=w42:T1)
                n177 = case shown="\"False\", Default" w36 {
                  tunnel: w42 -> [w57 _]
                  tunnel: w36 -> [w56 _]
                  tunnel: w41 -> [w55 w250]
                  tunnel: w40 -> [w54 w251]
                  tunnel: w39 -> [w53 _]
                  tunnel: [w52 FALSE] -> w38
                  tunnel: [w50 w249] -> w37
                  frame "False", Default {
                    n178 = property on="status TF" class="Bool (strict)"("Blinking"=TRUE) -> (error out=w45:errorcluster)  [unwired: 2 in, 1 out]
                    n179 = case shown="\"Button Messwerte\"" w56 {
                      tunnel: w57 -> [_ _ w65 w73 w81 w89 w97 w105 w114 w122 w130 w138 w146 w154 w163 w171 w179 w187 w195 w203 w211 w219 w226 w234 w243]
                      tunnel: w55 -> [w58 w61 _ _ _ _ _ _ _ _ _ _ _ _ _ _ _ _ _ _ _ _ _ _ _]
                      tunnel: [w58 w61 w63 w71 w78 w86 w94 w103 w110 w120 w127 w135 w144 w152 w160 w169 w177 w184 w192 w200 w209 w217 w224 w232 w239] -> w51
                      tunnel: w54 -> [_ _ w66 w74 w82 w90 w98 w106 w115 w123 w131 w139 w147 w155 w164 w172 w180 w188 w196 w204 w212 w220 w227 w235 w244]
                      tunnel: w53 -> [_ _ w64 w72 w80 w88 w96 w104 w113 w121 w129 w137 w145 w153 w162 w170 w178 w186 w194 w202 w210 w218 w225 w233 w242]
                      tunnel: [_ TRUE _ _ _ _ _ _ _ _ _ _ _ _ _ _ _ _ _ _ _ _ _ _ _] -> w52
                      tunnel: w45 -> [_ w59 _ _ _ _ _ _ _ _ _ _ _ _ _ _ _ _ _ _ _ _ _ _ _]
                      tunnel: [_ w59 _ _ _ _ _ _ _ _ _ _ _ _ _ _ _ _ _ _ _ _ _ _ _] -> w44
                      frame Default {
                      }
                      frame "Stop" {
                      }
                      frame "Button AC_DC" {
                        n180 = property on="status abc" class="Str"("Value"="executing  \"AC_DC\"" ("status abc")) -> ()  [unwired: 2 in, 2 out]
                        n181 = call "BaseProcess.call process 1.vi"("i ref in"=w66, "Object"=w64, "Selector"="SetAC_DC", "CallType"=enum16{"simple", "synchronous", "asynchronous"}."synchronous", "Data"=w65, "Data Descriptor"="S:1") -> ("error out"=w63:errorcluster)  [unwired: 11 in, 2 out]
                      }
                      frame "Button Peak" {
                        n182 = property on="status abc" class="Str"("Value"="executing  \"Peak\"" ("status abc")) -> ()  [unwired: 2 in, 2 out]
                        n183 = call "BaseProcess.call process 1.vi"("i ref in"=w74, "Object"=w72, "Selector"="SetPeak", "CallType"=enum16{"simple", "synchronous", "asynchronous"}."synchronous", "Data"=w73, "Data Descriptor"="S:1") -> ("error out"=w71:errorcluster)  [unwired: 11 in, 2 out]
                      }
                      frame "Set_Rel" {
                        n184 = property on="status abc" class="Str"("Value"="executing  \"set Relative value\"" ("status abc")) -> ()  [unwired: 2 in, 2 out]
                        n185 = call "BaseProcess.call process 1.vi"("i ref in"=w82, "Object"=w80, "Selector"="SetRelValue", "CallType"=enum16{"simple", "synchronous", "asynchronous"}."synchronous", "Data"=w81, "Data Descriptor"="S:1") -> ("error out"=w78:errorcluster)  [unwired: 11 in, 2 out]
                      }
                      frame "Set_lower" {
                        n186 = property on="status abc" class="Str"("Value"="executing  \"set lower\"" ("status abc")) -> ()  [unwired: 2 in, 2 out]
                        n187 = call "BaseProcess.call process 1.vi"("i ref in"=w90, "Object"=w88, "Selector"="SetLower", "CallType"=enum16{"simple", "synchronous", "asynchronous"}."synchronous", "Data"=w89, "Data Descriptor"="S:1") -> ("error out"=w86:errorcluster)  [unwired: 11 in, 2 out]
                      }
                      frame "Set_upper" {
                        n188 = property on="status abc" class="Str"("Value"="executing  \"set upper\"" ("status abc")) -> ()  [unwired: 2 in, 2 out]
                        n189 = call "BaseProcess.call process 1.vi"("i ref in"=w98, "Object"=w96, "Selector"="SetUpper", "CallType"=enum16{"simple", "synchronous", "asynchronous"}."synchronous", "Data"=w97, "Data Descriptor"="S:1") -> ("error out"=w94:errorcluster)  [unwired: 11 in, 2 out]
                      }
                      frame "Button Limit" {
                        n190 = property on="status abc" class="Str"("Value"="executing  \"Limit\"" ("status abc")) -> ()  [unwired: 2 in, 2 out]
                        n191 = call "BaseProcess.call process 1.vi"("i ref in"=w106, "Object"=w104, "Selector"="SetLimit", "CallType"=enum16{"simple", "synchronous", "asynchronous"}."synchronous", "Data"=w105, "Data Descriptor"="S:1") -> ("error out"=w103:errorcluster)  [unwired: 11 in, 2 out]
                      }
                      frame "Button Messwerte" {
                        n192 = property on="status abc" class="Str"("Value"="executing  \"Messwerte\"" ("status abc")) -> ()  [unwired: 2 in, 2 out]
                        n193 = call "BaseProcess.call process 1.vi"("i ref in"=w115, "Object"=w113, "Selector"="Messwerte", "CallType"=enum16{"simple", "synchronous", "asynchronous"}."synchronous", "Data"=w114, "Data Descriptor"="S:1", "timeout (ms)"=100000) -> ("error out"=w110:errorcluster)  [unwired: 10 in, 2 out]
                      }
                      frame "Button Filter" {
                        n194 = property on="status abc" class="Str"("Value"="executing  \"Filter\"" ("status abc")) -> ()  [unwired: 2 in, 2 out]
                        n195 = call "BaseProcess.call process 1.vi"("i ref in"=w123, "Object"=w121, "Selector"="SetFilter", "CallType"=enum16{"simple", "synchronous", "asynchronous"}."synchronous", "Data"=w122, "Data Descriptor"="S:1") -> ("error out"=w120:errorcluster)  [unwired: 11 in, 2 out]
                      }
                      frame "Button Auto_Range" {
                        n196 = property on="status abc" class="Str"("Value"="executing  \"Auto Range\"" ("status abc")) -> ()  [unwired: 2 in, 2 out]
                        n197 = call "BaseProcess.call process 1.vi"("i ref in"=w131, "Object"=w129, "Selector"="SetAutoRange", "CallType"=enum16{"simple", "synchronous", "asynchronous"}."synchronous", "Data"=w130, "Data Descriptor"="S:1") -> ("error out"=w127:errorcluster)  [unwired: 11 in, 2 out]
                      }
                      frame "Button Rel" {
                        n198 = property on="status abc" class="Str"("Value"="executing  \"Relative\"" ("status abc")) -> ()  [unwired: 2 in, 2 out]
                        n199 = call "BaseProcess.call process 1.vi"("i ref in"=w139, "Object"=w137, "Selector"="SetRel", "CallType"=enum16{"simple", "synchronous", "asynchronous"}."synchronous", "Data"=w138, "Data Descriptor"="S:1") -> ("error out"=w135:errorcluster)  [unwired: 11 in, 2 out]
                      }
                      frame "Button CField" {
                        n200 = property on="status abc" class="Str"("Value"="executing  \"CField\"" ("status abc")) -> ()  [unwired: 2 in, 2 out]
                        n201 = call "BaseProcess.call process 1.vi"("i ref in"=w147, "Object"=w145, "Selector"="SetCField", "CallType"=enum16{"simple", "synchronous", "asynchronous"}."synchronous", "Data"=w146, "Data Descriptor"="S:1") -> ("error out"=w144:errorcluster)  [unwired: 11 in, 2 out]
                      }
                      frame "Button CTemp" {
                        n202 = property on="status abc" class="Str"("Value"="executing  \"CTemp\"" ("status abc")) -> ()  [unwired: 2 in, 2 out]
                        n203 = call "BaseProcess.call process 1.vi"("i ref in"=w155, "Object"=w153, "Selector"="SetCTemp", "CallType"=enum16{"simple", "synchronous", "asynchronous"}."synchronous", "Data"=w154, "Data Descriptor"="S:1") -> ("error out"=w152:errorcluster)  [unwired: 11 in, 2 out]
                      }
                      frame "Button Zero" {
                        n204 = property on="status abc" class="Str"("Value"="executing  \"Zero\"" ("status abc")) -> ()  [unwired: 2 in, 2 out]
                        n205 = call "BaseProcess.call process 1.vi"("i ref in"=w164, "Object"=w162, "Selector"="Zero", "CallType"=enum16{"simple", "synchronous", "asynchronous"}."synchronous", "Data"=w163, "Data Descriptor"="S:1", "timeout (ms)"=100000) -> ("error out"=w160:errorcluster)  [unwired: 10 in, 2 out]
                      }
                      frame "Button Reset" {
                        n206 = property on="status abc" class="Str"("Value"="executing  \"Reset\"" ("status abc")) -> ()  [unwired: 2 in, 2 out]
                        n207 = call "BaseProcess.call process 1.vi"("i ref in"=w172, "Object"=w170, "Selector"="Reset", "CallType"=enum16{"simple", "synchronous", "asynchronous"}."synchronous", "Data"=w171, "Data Descriptor"="S:1") -> ("error out"=w169:errorcluster)  [unwired: 11 in, 2 out]
                      }
                      frame "Button Local" {
                        n208 = property on="status abc" class="Str"("Value"="executing  \"Local\"" ("status abc")) -> ()  [unwired: 2 in, 2 out]
                        n209 = call "BaseProcess.call process 1.vi"("i ref in"=w180, "Object"=w178, "Selector"="SetLocal", "CallType"=enum16{"simple", "synchronous", "asynchronous"}."synchronous", "Data"=w179, "Data Descriptor"="S:1") -> ("error out"=w177:errorcluster)  [unwired: 11 in, 2 out]
                      }
                      frame "Button Init" {
                        n210 = property on="status abc" class="Str"("Value"="executing  \"Init\"" ("status abc")) -> ()  [unwired: 2 in, 2 out]
                        n211 = call "BaseProcess.call process 1.vi"("i ref in"=w188, "Object"=w186, "Selector"="Init", "CallType"=enum16{"simple", "synchronous", "asynchronous"}."synchronous", "Data"=w187, "Data Descriptor"="S:1") -> ("error out"=w184:errorcluster)  [unwired: 11 in, 2 out]
                      }
                      frame "Enum Unit" {
                        n212 = property on="status abc" class="Str"("Value"="executing  \"Unit\"" ("status abc")) -> ()  [unwired: 2 in, 2 out]
                        n213 = call "BaseProcess.call process 1.vi"("i ref in"=w196, "Object"=w194, "Selector"="SetUnit", "CallType"=enum16{"simple", "synchronous", "asynchronous"}."synchronous", "Data"=w195, "Data Descriptor"="S:1") -> ("error out"=w192:errorcluster)  [unwired: 11 in, 2 out]
                      }
                      frame "Enum Range" {
                        n214 = property on="status abc" class="Str"("Value"="executing  \"Range\"" ("status abc")) -> ()  [unwired: 2 in, 2 out]
                        n215 = call "BaseProcess.call process 1.vi"("i ref in"=w204, "Object"=w202, "Selector"="SetRange", "CallType"=enum16{"simple", "synchronous", "asynchronous"}."synchronous", "Data"=w203, "Data Descriptor"="S:1") -> ("error out"=w200:errorcluster)  [unwired: 11 in, 2 out]
                      }
                      frame "Enum Max" {
                        n216 = property on="status abc" class="Str"("Value"="executing  \"Max\"" ("status abc")) -> ()  [unwired: 2 in, 2 out]
                        n217 = call "BaseProcess.call process 1.vi"("i ref in"=w212, "Object"=w210, "Selector"="SetMax", "CallType"=enum16{"simple", "synchronous", "asynchronous"}."synchronous", "Data"=w211, "Data Descriptor"="S:1") -> ("error out"=w209:errorcluster)  [unwired: 11 in, 2 out]
                      }
                      frame "Enum Temp" {
                        n218 = property on="status abc" class="Str"("Value"="executing  \"Temp\"" ("status abc")) -> ()  [unwired: 2 in, 2 out]
                        n219 = call "BaseProcess.call process 1.vi"("i ref in"=w220, "Object"=w218, "Selector"="SetTemp", "CallType"=enum16{"simple", "synchronous", "asynchronous"}."synchronous", "Data"=w219, "Data Descriptor"="S:1") -> ("error out"=w217:errorcluster)  [unwired: 11 in, 2 out]
                      }
                      frame "Button OK" {
                        n220 = call "BaseProcess.call process 1.vi"("i ref in"=w227, "Object"=w225, "Selector"="OK", "CallType"=enum16{"simple", "synchronous", "asynchronous"}."synchronous", "Data"=w226, "Data Descriptor"="S:1") -> ("error out"=w224:errorcluster)  [unwired: 11 in, 2 out]
                      }
                      frame "SaveSettings" {
                        n221 = property on="status abc" class="Str"("Value"="executing  \"save settings\"" ("status abc")) -> ()  [unwired: 2 in, 2 out]
                        n222 = call "BaseProcess.call process 1.vi"("i ref in"=w235, "Object"=w233, "Selector"="SaveSettings", "CallType"=enum16{"simple", "synchronous", "asynchronous"}."synchronous", "Data"=w234, "Data Descriptor"="C:N") -> ("error out"=w232:errorcluster)  [unwired: 11 in, 2 out]
                      }
                      frame "LoadSettings" {
                        n223 = property on="status abc" class="Str"("Value"="executing  \"load settings\"" ("status abc")) -> ()  [unwired: 2 in, 2 out]
                        n224 = call "BaseProcess.call process 1.vi"("i ref in"=w244, "Object"=w242, "Selector"="LoadSettings", "CallType"=enum16{"simple", "synchronous", "asynchronous"}."synchronous", "Data"=w243, "Data Descriptor"="C:N", "timeout (ms)"=50000) -> ("error out"=w239:errorcluster)  [unwired: 10 in, 2 out]
                      }
                    }
                    n225 = property on="Lesen" class="Bool (strict)"(error in=w51) -> (error out=w47:errorcluster, "Value"=w48:bool)  [unwired: 1 in, 1 out]
                    n226 = property on="status TF" class="Bool (strict)"(error in=w44, "Blinking"=FALSE) -> ()  [unwired: 1 in, 2 out]
                    n227 = property on="Lesen" class="Bool (strict)"(error in=w47, "Val(Sgnl)"=w48) -> (error out=w50:errorcluster)  [unwired: 1 in, 1 out]
                  }
                  frame "Lesen" {
                    n228 = call "CSGaussmeter.get data to modify.vi"("i ref in"=w251, "error in (no error)"=w250) -> ("i ref out"=w255:refnum<vi>, "i attribute"=w257:T12, "timed out"=w256:bool, "error out"=w253:errorcluster)  [unwired: 14 in]
                    n229 = case shown="False" w256 {
                      tunnel: w257 -> [w261 _]
                      tunnel: [w260 w264] -> w254
                      tunnel: w255 -> [w260 w264]
                      tunnel: w253 -> [w259 w263]
                      tunnel: [w259 w263] -> w252
                      frame False {
                        n230 = Unbundle By Name(w261) -> ("actValues"=w258:T14, "Messwerte 2"=→"Messwerte 2":string)
                        n231 = property on="Control" class="Clust (strict)"("Value"=w258) -> ()  [unwired: 2 in, 2 out]
                      }
                      frame True {
                      }
                    }
                    n232 = call "CSObj.release.vi"("i ref in"=w254, "error in (no error)"=w252) -> ("error out"=w249:errorcluster)  [unwired: 16 in, 1 out]
                  }
                }
              }
              frame True {
                (unwired) errorcluster {"status"=FALSE, "code"=0, "source"=""} ("error out")
              }
            }
            n233 = Unbundle(w31) -> ("status"=w25:bool, "source"=w27:string)  [unwired: 1 out]
            n234 = Not(x=w25) -> (.not. x?=w24:bool)
            n235 = Select(t=w27, s=w25, f="No Error") -> (s? t:f=→"status abc":string)
            n236 = property on="status TF" class="Bool (strict)"("Value"=w24) -> ()  [unwired: 2 in, 2 out]
          }
        }
        frame #2 {
          n237 = Two Button Dialog(message="Save settings before closing?", 1:"No" ("F button name (\"Cancel\")"), 2:"Yes" ("T button name (\"OK\")")) -> (T button?=w504:bool)
          n238 = case "save settings?" shown="True" w504 {
            tunnel: w503 -> [_ w517]
            tunnel: w502 -> [w508 w516]
            tunnel: [w508 w509] -> w501
            frame False {
            }
            frame True {
              n239 = String To Path(string="F:\\LVSCC\\LV820\\GPL\\Projects\\cs-framework\\CSClass\\CSHitrap\\CSGaussmeter\\") -> (path=w512:path)
              n240 = File Dialog(7:"setting file" ("prompt"), 11:w512) -> (3:w514:path)  [unwired: 5 in, 3 out]
              n241 = Path To String(path=w514) -> (string=w511:string)
              n242 = call-poly "CoreLib.data 2 byte array.vi"("string"=w511) -> ("byteArray out"=w510:T1)  [unwired: 18 in]
              n243 = call "BaseProcess.call process 1.vi"("i ref in"=w517, "Selector"="SaveSettings", "CallType"=enum16{"simple", "synchronous", "asynchronous"}."synchronous", "Data"=w510, "error in (no error)"=w516, "Data Descriptor"="C:N") -> ("error out"=w509:errorcluster)  [unwired: 11 in, 2 out]
            }
          }
        }
      }
    }
    frame Error {
    }
  }
  "error out" <- w6
